vi "Post-Uninstall Custom Action.vi"(10 "Variant":variant) -> (0 "error out":errorcluster)   [LabVIEW 2015]
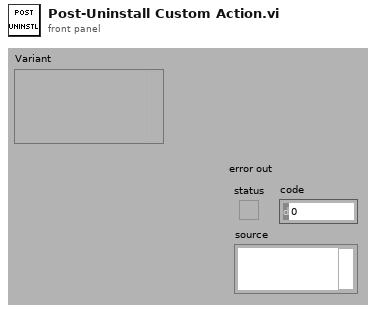
[diagram p1: front panel]
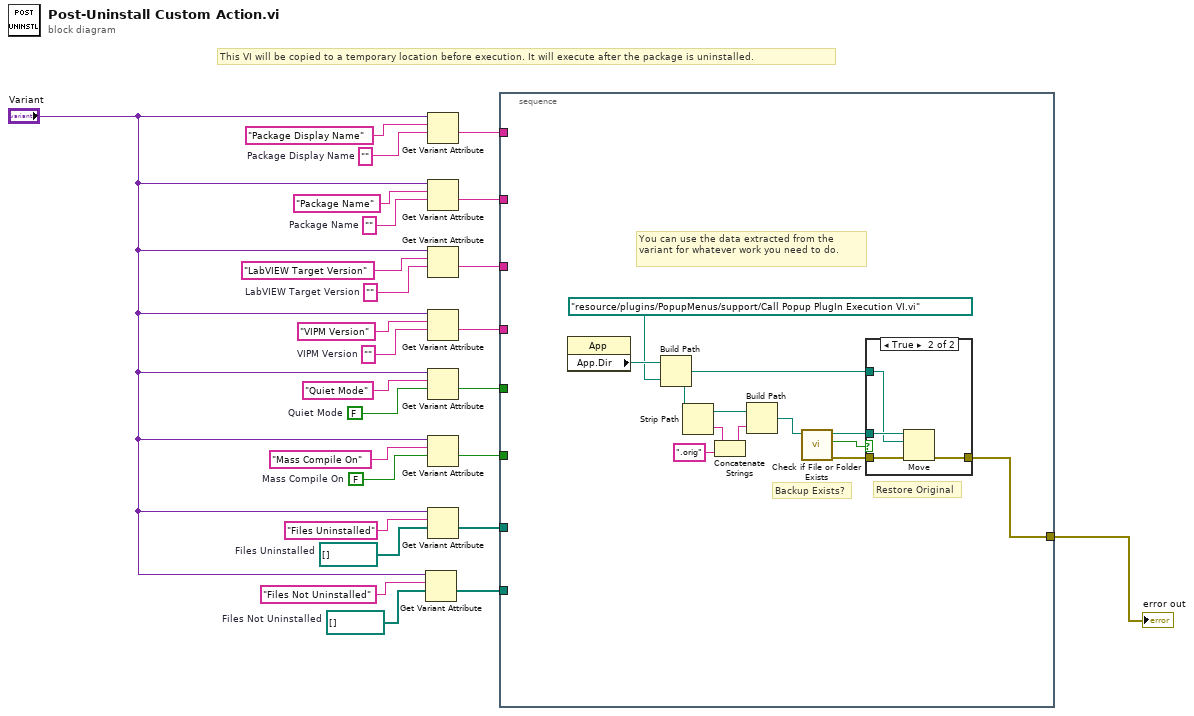
[diagram p0: block diagram]
diagram:
  w2 = path[] []  # Files Not Uninstalled
  w3 = path[] []  # Files Uninstalled
  w9 = FALSE  # Mass Compile On
  w10 = ""  # Package Display Name
  w17 = FALSE  # Quiet Mode
  w20 = ""  # VIPM Version
  w22 = ""  # LabVIEW Target Version
  w24 = ""  # Package Name
  # "This VI will be copied to a temporary location before execution. It will execute after the package is uninstalled."
  n1 = Get Variant Attribute(Variant="Variant", name="Files Not Uninstalled", default value (empty Variant)=w2) -> (value=w7:path[])  [unwired: 1 in, 3 out]
  n2 = Get Variant Attribute(Variant="Variant", name="Package Display Name", default value (empty Variant)=w10) -> (value=w16:string)  [unwired: 1 in, 3 out]
  n3 = Get Variant Attribute(Variant="Variant", name="Package Name", default value (empty Variant)=w24) -> (value=w15:string)  [unwired: 1 in, 3 out]
  n4 = Get Variant Attribute(Variant="Variant", name="LabVIEW Target Version", default value (empty Variant)=w22) -> (value=w14:string)  [unwired: 1 in, 3 out]
  n5 = Get Variant Attribute(Variant="Variant", name="VIPM Version", default value (empty Variant)=w20) -> (value=w13:string)  [unwired: 1 in, 3 out]
  n6 = Get Variant Attribute(Variant="Variant", name="Quiet Mode", default value (empty Variant)=w17) -> (value=w12:bool)  [unwired: 1 in, 3 out]
  n7 = Get Variant Attribute(Variant="Variant", name="Mass Compile On", default value (empty Variant)=w9) -> (value=w11:bool)  [unwired: 1 in, 3 out]
  n8 = Get Variant Attribute(Variant="Variant", name="Files Uninstalled", default value (empty Variant)=w3) -> (value=w6:path[])  [unwired: 1 in, 3 out]
  n9 = stacked-sequence {
    tunnel: w16 -> [_]
    tunnel: w15 -> [_]
    tunnel: w14 -> [_]
    tunnel: w13 -> [_]
    tunnel: w12 -> [_]
    tunnel: w11 -> [_]
    tunnel: w6 -> [_]
    tunnel: w7 -> [_]
    tunnel: [w27] -> w1
    frame #0 {
      # "Restore Original"
      # "Backup Exists?"
      # "You can use the data extracted from the variant for whatever work you need to do."
      n10 = property class="App"() -> ("App.Dir"=w38:path)  [unwired: 2 in, 2 out]
      n11 = Build Path(base path=w38, name or relative path=path "resource/plugins/PopupMenus/support/Call Popup PlugIn Execution VI.vi") -> (appended path=w29:path)
      n12 = Strip Path(path=w29) -> (stripped path=w36:path, name=w35:string)
      n13 = Concatenate Strings(w35, ".orig" ("string")) -> (w34:string)
      n14 = Build Path(base path=w36, name or relative path=w34) -> (appended path=w32:path)
      n15 = call <vilib>:"Check if File or Folder Exists.vi"("path"=w32) -> ("error out"=w28:errorcluster, "file or folder exists?"=w31:bool, "dup path"=w30:path)  [unwired: 8 in]
      n16 = case shown="True" w31 {
        tunnel: w30 -> [_ w43]
        tunnel: w29 -> [_ w42]
        tunnel: w28 -> [w39 w41]
        tunnel: [w39 w40] -> w27
        frame False {
        }
        frame True {
          n17 = Move(source path=w43, error in=w41, 10:w42) -> (error out=w40:errorcluster)  [unwired: 2 in, 2 out]
        }
      }
    }
  }
  "error out" <- w1
